vi "postData.vi"(7 "LabVIEW Web Service Request":refnum<class "Web Request.lvclass">) -> ()   [LabVIEW 2016]
uses:
  <vilib>/wsapi/Web Request.lvclass
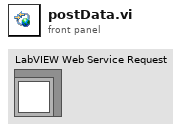
[diagram p1: front panel]
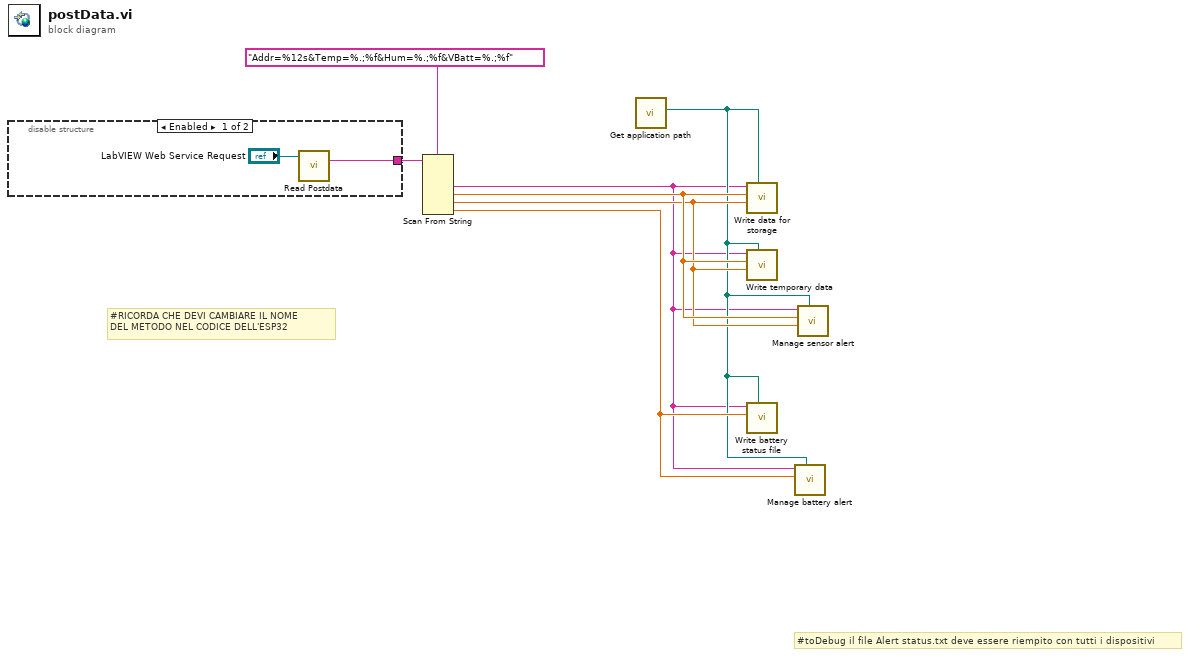
[diagram p0: block diagram]
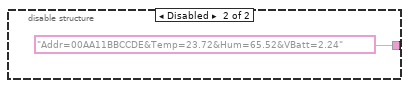
[diagram p2: hidden frame]
diagram:
  # "#toDebug il file Alert status.txt deve essere riempito con tutti i dispositivi"
  # "#RICORDA CHE DEVI CAMBIARE IL NOME\nDEL METODO NEL CODICE DELL'ESP32"
  n1 = disable-structure shown="Enabled" {
    disable-tunnel: [w8 "Addr=00AA11BBCCDE&Temp=23.72&Hum=65.52&VBatt=2.24" ("input string")] -> w7
    frame Enabled {
      n2 = call <vilib>:"Read Postdata.vi"("LabVIEW Web Service Request"="LabVIEW Web Service Request") -> ("postdata"=w8:string)  [unwired: 12 in, 2 out]
    }
    frame Disabled {
    }
  }
  n3 = Scan From String(format string="Addr=%12s&Temp=%.;%f&Hum=%.;%f&VBatt=%.;%f", input string=w7) -> (output 1=w2:string, output 2=w6:dbl, output 3=w5:dbl, output 4=w4:dbl)  [unwired: 6 in, 3 out]
  n4 = call "Get application path.vi"() -> ("Application path"=w3:path)  [unwired: 11 in]
  n5 = call "Write data for storage.vi"("Application path"=w3, "Humidity"=w5, "Temperature"=w6, "MAC address"=w2) -> ()  [unwired: 6 in, 2 out]
  n6 = call "Write temporary data.vi"("Application path"=w3, "Humidity"=w5, "Temperature"=w6, "MAC address"=w2) -> ()  [unwired: 6 in, 2 out]
  n7 = call "Write battery status file.vi"("Application path"=w3, "Battery voltage"=w4, "MAC address"=w2) -> ()  [unwired: 7 in, 2 out]
  n8 = call "Manage battery alert.vi"("Application path"=w3, "Vbattery"=w4, "MAC address"=w2) -> ()  [unwired: 8 in, 1 out]
  n9 = call "Manage sensor alert.vi"("Application path"=w3, "Humidity"=w5, "Temperature"=w6, "MAC address"=w2) -> ()  [unwired: 7 in, 1 out]
